vi "Compatibility Trigger Drive.vi"() -> ()   [LabVIEW 2023]
doc: "The Compatibility Trigger Drive example demonstrates how to drive a signal on a trigger line. A high-level grab is used as the acquisition type. <B>IMAQdx Compatability Trigger Drive2</B> outputs a signal on an external or RTSI trigger line.\n\nThis example uses the IMAQdx driver to interface with a Camera Link frame grabber. It uses the NI-IMAQdx Compatibility for NI-IMAQ API to facilitate migration between the two drivers. The NI-IMAQdx VIs are drop-in replacements to existing NI-IMAQ VIs."
uses:
  <vilib>/vision/driver/NI_Vision_Acquisition_Software.lvlib
panel:
  in  "Trigger drive":u32(ring)=6 items=["Disabled", "Acquisition in Progress", "Acquisition Done", "Pixel Clock", "Unasserted", "Asserted", "Horizontal Synchronization Signal", "Vertical Synchronization Signal", "Frame Start", "Frame Done", "Scaled Encoder"]
  in  "Camera Name":refnum<k21> caption="IMAQdx Session"
  in  "Trigger Polarity":u32(ring) items=["High True", "Low True"]
  in  "Trigger Type":u32(ring) items=["External"=0, "RTSI"=1, "ISO Out"=3]
  in  "Trigger Number":u32
  in  "Stop":bool
  out "Image":T1(plugin-control)
  # "Overview: Demonstrates how to drive an internal signal on an external trigger or RTSI line.\nRequirements: Vision Acquisition Software 18.0 or later, PCIe-1427, PCIe-1433, PXIe-1435, or PCIe-1437 frame grabber.\nInstructions: \n1. Select the IMAQdx Camera Name.\n2. Run the VI."
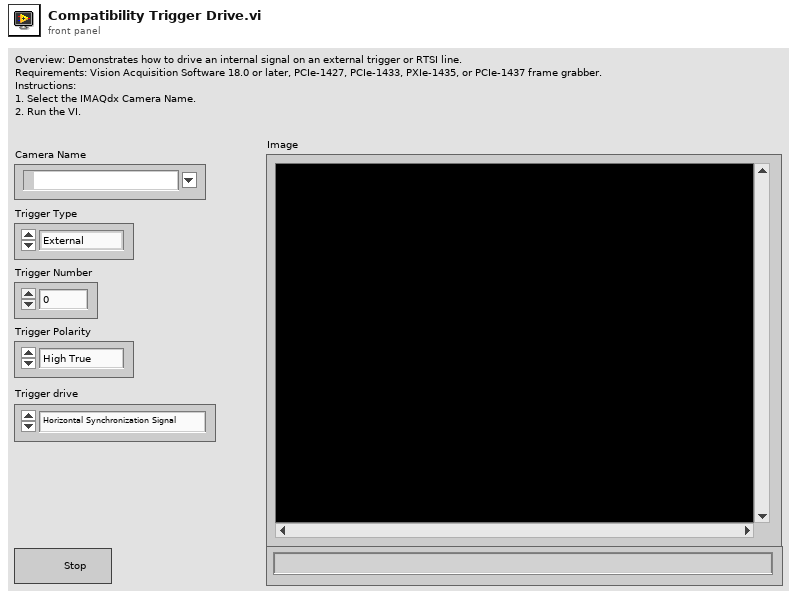
[diagram p1: front panel]
types:
  T1 = typedef "IMAQ Image.ctl" = refnum<image>
  T2 = typedef "IMAQdx.ctl" = refnum<k21>
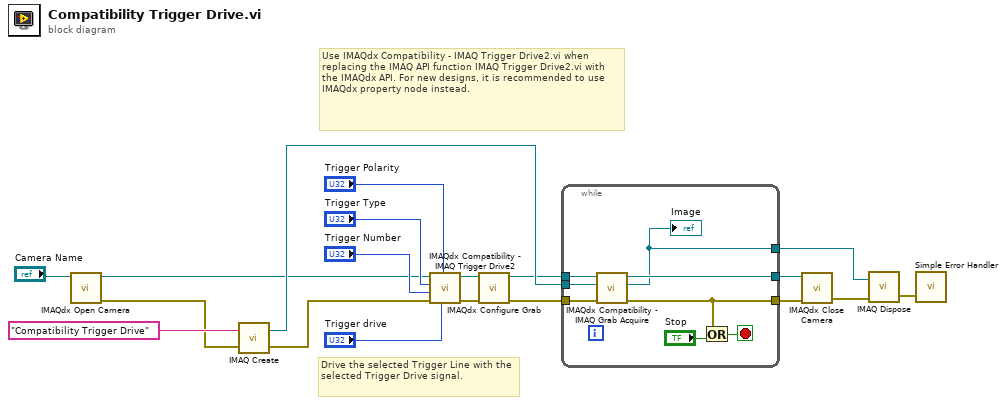
[diagram p0: block diagram]
diagram:
  # "Use IMAQdx Compatibility - IMAQ Trigger Drive2.vi when replacing the IMAQ API function IMAQ Trigger Drive2.vi with the IMAQdx API. For new designs, it is recommended to use IMAQdx property node instead."
  # "Drive the selected Trigger Line with the selected Trigger Drive signal."
  n1 = call <vilib>:"IMAQdx Open Camera.vi"("Session In"="Camera Name") -> ("error out"=w8:errorcluster, "Session Out"=w7:T2)  [unwired: 9 in]
  n2 = call "IMAQ Create"("Image Name"="Compatibility Trigger Drive", "error in (no error)"=w8) -> ("New Image"=w12:T1, "error out"=w10:errorcluster)  [unwired: 2 in, 1 out]
  n3 = call <vilib>:"IMAQdx Compatibility - IMAQ Trigger Drive2.vi"("Trigger drive"="Trigger drive", "Trigger polarity"="Trigger Polarity", "error in (no error)"=w10, "Trigger Number"="Trigger Number", "Trigger Type"="Trigger Type", "Session In"=w7) -> ("error out"=w6:errorcluster, "Session Out"=w5:T2)  [unwired: 4 in]
  n4 = call <vilib>:"IMAQdx Configure Grab.vi"("error in"=w6, "Session In"=w5) -> ("error out"=w4:errorcluster, "Session Out"=w3:T2)  [unwired: 8 in]
  n5 = while {
    tunnel: w12 -> [w23]
    tunnel: w4 -> [w24]
    tunnel: w3 -> [w25]
    tunnel: [w22] -> w18
    tunnel: [w21] -> w17
    tunnel: [w20] -> w9
    stop <- w27 stop-if-true
    n6 = call <vilib>:"IMAQdx Compatibility - IMAQ Grab Acquire.vi"("error in (no error)"=w24, "Image In"=w23, "Session In"=w25) -> ("error out"=w21:errorcluster, "Image Out"=w20:T1, "Session Out"=w22:T2)  [unwired: 5 in, 1 out]
    "Image" <- w20
    n7 = Or(x=w21, y="Stop") -> (x .or. y?=w27:bool)
  }
  n8 = call <vilib>:"IMAQdx Close Camera.vi"("error in"=w17, "Session In"=w18) -> ("error out"=w11:errorcluster)  [unwired: 9 in]
  n9 = call "IMAQ Dispose"("Image"=w9, "error in (no error)"=w11) -> ("error out"=w19:errorcluster)  [unwired: 1 in, 3 out]
  n10 = call <vilib>:"Simple Error Handler.vi"("error in (no error)"=w19) -> ()  [unwired: 1 in, 8 out]
